vi "proccessPacket.vi"(8 "error in (no error)":errorcluster, 10 "tcp packet":string, 11 "tcpServer in":refnum<class "TcpServer.lvclass">) -> (0 "error out":errorcluster, 3 "tcpServer out":refnum<class "TcpServer.lvclass">)   [LabVIEW 2018, in "TcpServer.lvclass"]
doc: "Receive json packet, procces it , check rules, \nsend the Ack to client and send user event to\nUser."
uses:
  TcpServer.lvclass
  TcpServer.lvclass/TcpServer.ctl
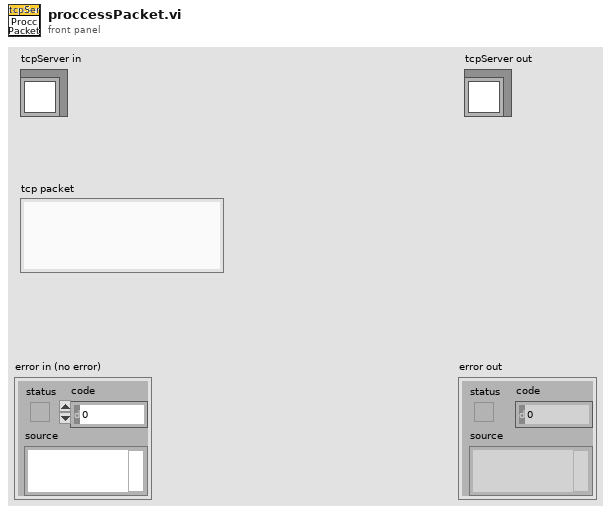
[diagram p1: front panel]
types:
  T1 = typedef "TcpServer.lvclass/userEventsTypeDef.ctl" = cluster{"TcpServer":refnum<user-event>, "Command":refnum<user-event>, "Ack":refnum<user-event>, "Event":refnum<user-event>, "Telemetry":refnum<user-event>}
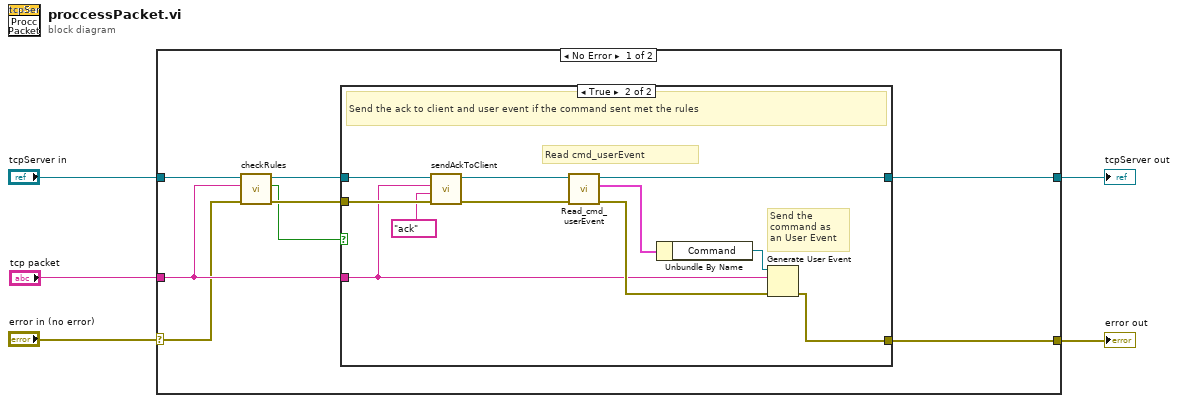
[diagram p0: block diagram]
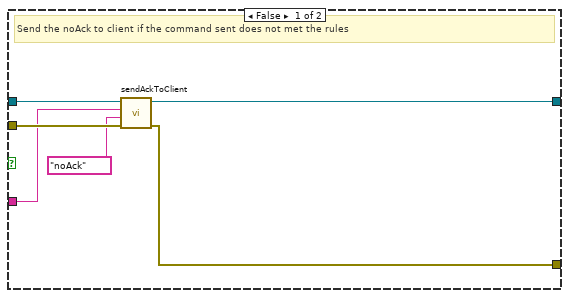
[diagram p2: hidden frame]
diagram:
  n1 = case shown="No Error" "error in (no error)" {
    selector: "error in (no error)" -> [w9 w32]
    tunnel: [w13 w32] -> w4
    tunnel: [w12 w31] -> w2
    tunnel: "tcpServer in" -> [w11 w31]
    tunnel: "tcp packet" -> [w10 _]
    frame No Error {
      n2 = call "checkRules.vi"("error in (no error)"=w9, "tcp packet"=w10, "tcpServer in"=w11) -> ("error out"=w7:errorcluster, "is ok?"=w6:bool, "tcpServer out"=w8:refnum<class "TcpServer.lvclass">)  [unwired: 6 in]
      n3 = case shown="True" w6 {
        tunnel: [w16 w30] -> w13
        tunnel: [w17 w29] -> w12
        tunnel: w10 -> [w15 w21]
        tunnel: w8 -> [w19 w23]
        tunnel: w7 -> [w18 w22]
        frame False {
          # "Send the noAck to client if the command sent does not met the rules"
          n4 = call "sendAckToClient.vi"("error in (no error)"=w18, "cmdStatus"="noAck", "Ack"=w15, "tcpServer in"=w19) -> ("error out"=w16:errorcluster, "tcpServer out"=w17:refnum<class "TcpServer.lvclass">)  [unwired: 6 in]
        }
        frame True {
          # "Read cmd_userEvent"
          # "Send the \ncommand as\nan User Event"
          # "Send the ack to client and user event if the command sent met the rules"
          n5 = call "sendAckToClient.vi"("error in (no error)"=w22, "cmdStatus"="ack", "Ack"=w21, "tcpServer in"=w23) -> ("error out"=w25:errorcluster, "tcpServer out"=w26:refnum<class "TcpServer.lvclass">)  [unwired: 6 in]
          n6 = call "Read_cmd_userEvent.vi"("error in (no error)"=w25, "tcpServer in"=w26) -> ("error out"=w24:errorcluster, "UserEvents"=w28:T1, "tcpServer out"=w29:refnum<class "TcpServer.lvclass">)  [unwired: 7 in]
          n7 = Unbundle By Name(w28) -> ("Command"=w27:refnum<user-event>)
          n8 = Generate User Event(user event=w27, event data cluster=w21, error in=w24) -> (error out=w30:errorcluster)  [unwired: 1 in, 1 out]
        }
      }
    }
    frame Error {
    }
  }
  "error out" <- w4
  "tcpServer out" <- w2
